vi "Zynq-Adder.vi"(10 "B_in_u8":u8, 11 "A_in_u8":u8) -> (3 "Sum_out_u8":u8)   [LabVIEW 2020]
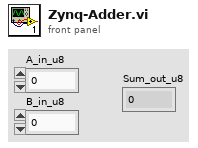
[diagram p1: front panel]
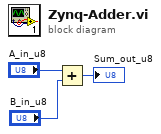
[diagram p0: block diagram]
diagram:
  n1 = Add(x="A_in_u8", y="B_in_u8") -> (x+y=→"Sum_out_u8":u8)
